vi "Get SMO Public API.vi"(8 "error in (no error)":errorcluster, 11 "instrument.PPMS in":refnum<class "instrument.PPMS.lvclass">) -> (0 "error out":errorcluster, 2 "Commands":string[](array[string]), 3 "instrument.PPMS out":refnum<class "instrument.PPMS.lvclass">)   [LabVIEW 2019, in "instrument.PPMS.lvclass"]
uses:
  instrument.PPMS.lvclass
  <userlib>/_OpenG.lib/array/array.llb/Delete Elements from 1D Array (String)__ogtk.vi
  <userlib>/LevyLab/Instrument Framework/Instrument Types/Cryostat/Instrument.Cryostat.lvclass
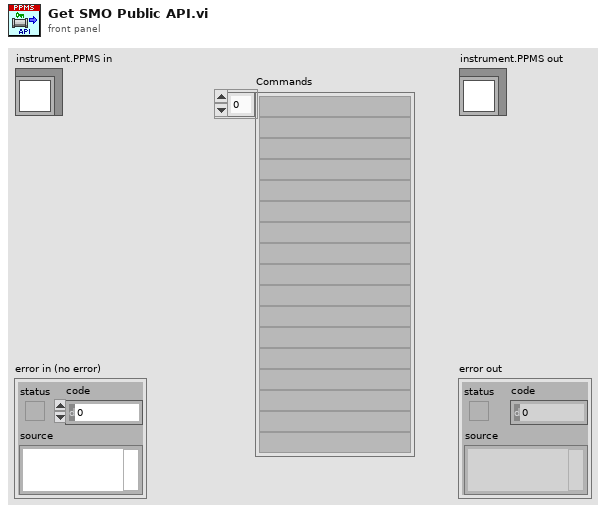
[diagram p1: front panel]
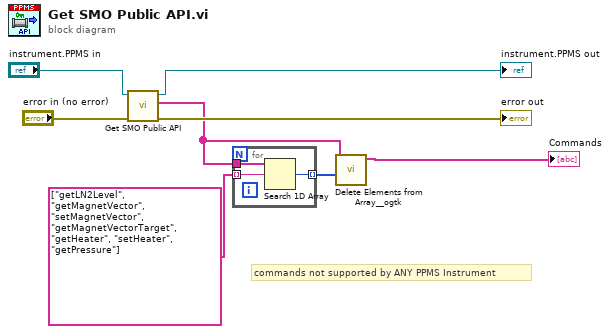
[diagram p0: block diagram]
diagram:
  # "commands not supported by ANY PPMS Instrument"
  n1 = call-parent "Get SMO Public API.vi"("error in (no error)"="error in (no error)", "Instrument.Cryostat in"="instrument.PPMS in") -> ("error out"=→"error out":errorcluster, "commands"=w2:string[], "Instrument.Cryostat out"=→"instrument.PPMS out":refnum<class "instrument.PPMS.lvclass">)  [unwired: 7 in]
  n2 = for {
    tunnel: [w11] -> w4 mode=indexing
    tunnel: string[] ["getLN2Level", "getMagnetVector", "setMagnetVector", "getMagnetVectorTarget", "getHeater", "setHeater", "getPressure"] ("Commands 2") -> [w10] mode=indexing
    tunnel: w2 -> [w9]
    n3 = Search 1D Array(1D array=w9, element=w10) -> (index of element=w11:i32)  [unwired: 1 in]
  }
  n4 = call-poly <userlib>:"Delete Elements from Array__ogtk.vi"("indices"=w4, "array"=w2) -> ("array w/ subset deleted"=→"Commands":string[])  [unwired: 8 in, 1 out]
